vi "Read Type.vi"(8 "error in (no error)":errorcluster, 11 "BC.lvclass in":refnum<class "NI_BC.lvclass">) -> (0 "error out":errorcluster, 2 "BC type":T1 items=["Dirichlet", "Neumann"], 3 "BC.lvclass out":refnum<class "NI_BC.lvclass">)   [LabVIEW 2017, in "NI_PDE.lvlib" / "NI_BC.lvclass"]
uses:
  <vilib>/gmath/pde.llb/BCClass/NI_BC.lvclass
  <vilib>/gmath/pde.llb/Common/PDE_BC Type.ctl
  <vilib>/gmath/pde.llb/BCClass/NI_BC.lvclass/NI_BC.ctl
  <vilib>/gmath/NI_PDE.lvlib
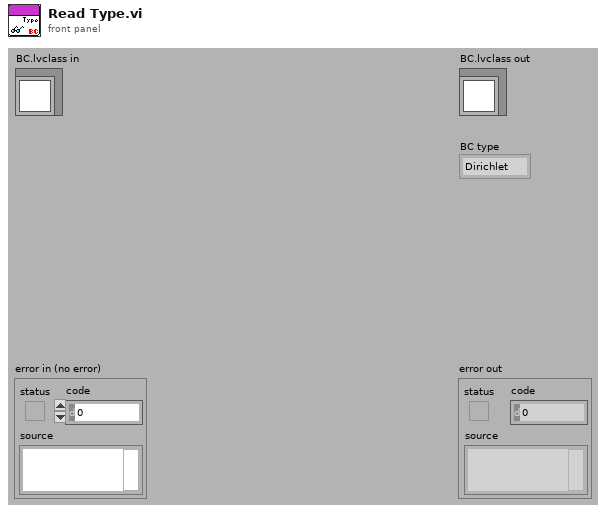
[diagram p1: front panel]
types:
  T1 = typedef "NI_PDE.lvlib/PDE_BC Type.ctl" = i32
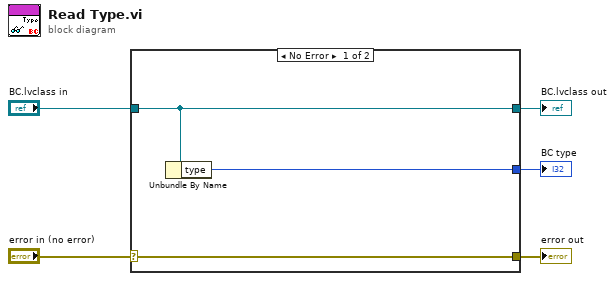
[diagram p0: block diagram]
diagram:
  n1 = case shown="No Error" "error in (no error)" {
    selector: "error in (no error)" -> [w8 w9]
    tunnel: [w8 w9] -> w4
    tunnel: [w7 w10] -> w2
    tunnel: "BC.lvclass in" -> [w7 w10]
    tunnel: [w6 _] -> w1
    frame No Error {
      n2 = Unbundle By Name(w7) -> ("type"=w6:T1)
    }
    frame Error {
    }
  }
  "error out" <- w4
  "BC.lvclass out" <- w2
  "BC type" <- w1
